vi "SbigClose.vi"(0 "error in":errorcluster, 2 "Sbig infos":T1[](array[typedef])) -> (3 "error out":errorcluster)   [LabVIEW 2009]
uses:
  Controls/SbigReference.ctl
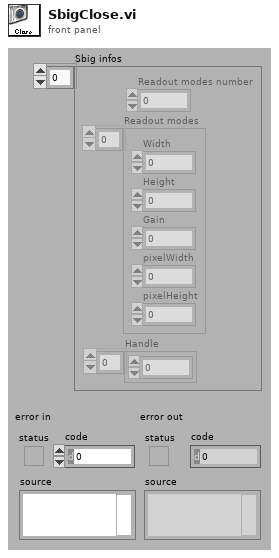
[diagram p1: front panel]
types:
  T1 = typedef "SbigReference.ctl" = cluster{"Readout modes number":u16, "Readout modes":cluster{"Width":u16, "Height":u16, "Gain":dbl, "pixelWidth":dbl, "pixelHeight":dbl}[], "Handle":u16[]}
  T2 = enum16{"0-NoCommand", "1-StartExposure", "2-EndExposure", "3-ReadoutLine", "4-DumpLines", "5-SetTemperatureRegulation", "6-QueryTemperatureStatus", "7-ActivateRelay", "8-PulseOut", "9-EstablishLink", "10-GetDriverInfo", "11-GetCCDInfo", "12-QueryCommandStatus", "13-MiscellaneousControl", "14-ReadSubstractLine", "15-UpdateClock", "16-ReadOffset", "17-OpenDriver", "18-CloseDriver", "19-TXSerialBytes", "20-GetSerialStatus", "21-AOTipTilt", "22-AOSetFocus", "23-AODelay", "24-GetTurboStatus", "25-EndReadout", "26-GetUSTimer", "27-OpenDevice", "28-CloseDevice", "29-SetIRQL", "30-GetIRQL", "31-GetLine", "32-GetLinkStatus", "33-GetDriverHandle", "34-SetDriverHandle", "35-StartReadout", "36-GetErrorString", "37-SetDriverControl", "38-GetDriverControl", "39-USBADControl", "40-QueryUSB", "41-GetPentiumCycleCount", "42-RWUSBI2C", "43-CFW"}
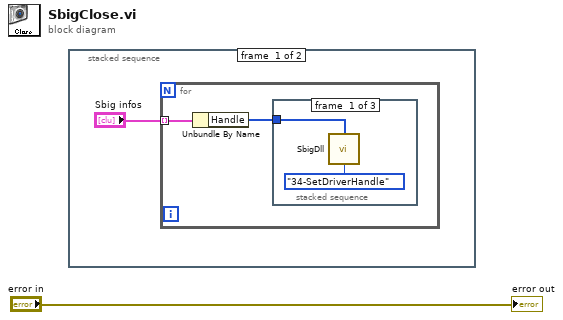
[diagram p0: block diagram]
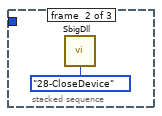
[diagram p2: hidden frame]
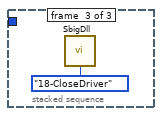
[diagram p3: hidden frame]
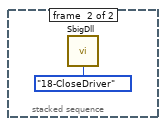
[diagram p4: hidden frame]
diagram:
  n1 = stacked-sequence {
    frame #0 {
      n2 = for {
        tunnel: "Sbig infos" -> [w4] mode=indexing
        n3 = Unbundle By Name(w4) -> ("Handle"=w3:u16[])
        n4 = stacked-sequence {
          tunnel: w3 -> [w5 _ _]
          frame #0 {
            n5 = call "SbigDll.vi"("Command"=T2."34-SetDriverHandle", "Parameters"=w5) -> ()  [unwired: 2 in, 4 out]
          }
          frame #1 {
            n6 = call "SbigDll.vi"("Command"=T2."28-CloseDevice") -> ()  [unwired: 3 in, 4 out]
          }
          frame #2 {
            n7 = call "SbigDll.vi"("Command"=T2."18-CloseDriver") -> ()  [unwired: 3 in, 4 out]
          }
        }
      }
    }
    frame #1 {
      n8 = call "SbigDll.vi"("Command"=T2."18-CloseDriver") -> ()  [unwired: 3 in, 4 out]
    }
  }
  "error out" <- "error in"
